vi "Data_2D_with_IgorX.vi"(6 "Data From Igor":bool, 8 "error in (no error)":errorcluster, 9 "Wave Name":string, 10 "Wave Prefix":string, 11 "2D Data IN":dbl[][](array[numeric])) -> (0 "error out":errorcluster, 2 "Wave Prefix Through":string, 3 "2D Data OUT":dbl[][](array[numeric]))   [LabVIEW 2014]
panel:
  in  "Igor Application IN":refnum<k7>
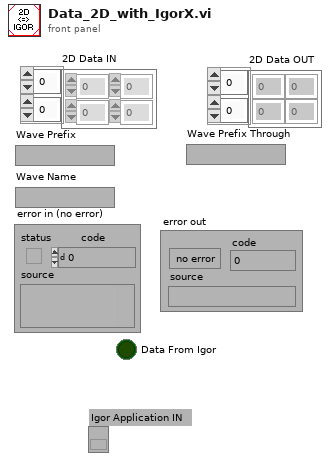
[diagram p1: front panel]
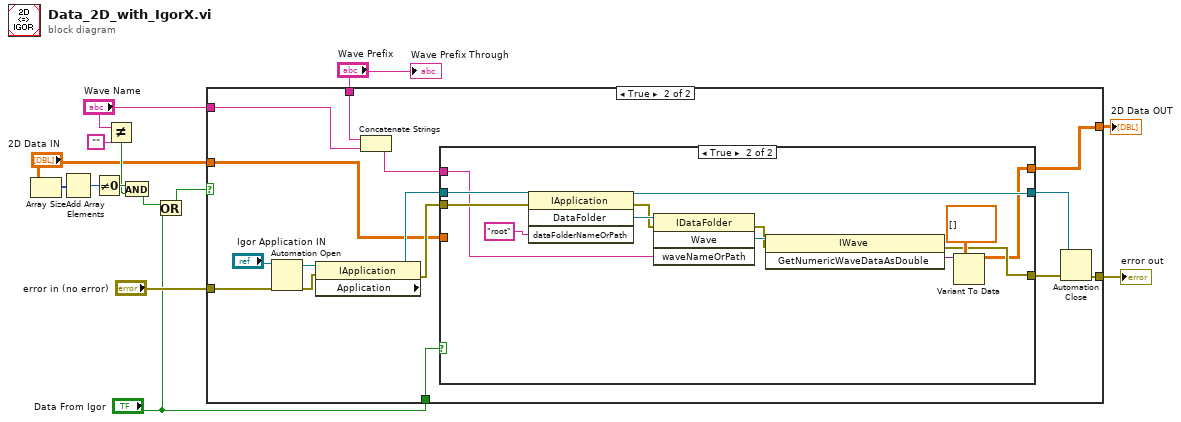
[diagram p0: block diagram]
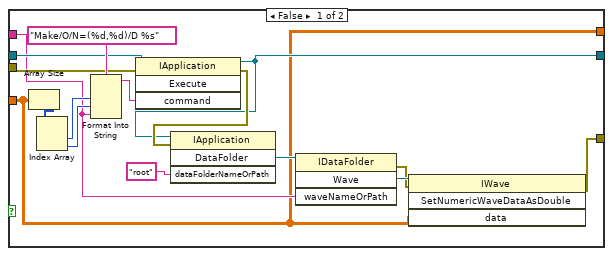
[diagram p3: hidden frame]
diagram:
  n1 = Array Size(array="2D Data IN") -> (size(s)=w14:i32[])
  n2 = Add Array Elements(numeric array=w14) -> (sum=w4:i32)
  n3 = Not Equal To 0?(x=w4) -> (x != 0?=w13:bool)
  n4 = Not Equal?(x="Wave Name", y="") -> (x != y?=w10:bool)
  n5 = And(x=w13, y=w10) -> (x .and. y?=w3:bool)
  n6 = Or(x=w3, y="Data From Igor") -> (x .or. y?=w1:bool)
  n7 = case shown="True" w1 {
    tunnel: "2D Data IN" -> [w15 w17]
    tunnel: "Wave Name" -> [_ w30]
    tunnel: "Wave Prefix" -> [_ w31]
    tunnel: "error in (no error)" -> [w16 w25]
    tunnel: [w16 w23] -> w8
    tunnel: "Data From Igor" -> [_ w29]
    tunnel: [w15 w18] -> w5
    frame False {
    }
    frame True {
      n8 = Automation Open(error in (no error)=w25, Automation Refnum="Igor Application IN") -> (Automation Refnum=w26:refnum<k7>, error out=w28:errorcluster)  [unwired: 2 in]
      n9 = property class="IApplication"(reference=w26, error in=w28) -> (error out=w24:errorcluster, "Application"=w22:refnum<k7>)  [unwired: 1 out]
      n10 = Concatenate Strings(w31, w30) -> (w20:string)
      n11 = case shown="True" w29 {
        tunnel: w24 -> [w45 w53]
        tunnel: [w37 w49] -> w21
        tunnel: w22 -> [w46 w52]
        tunnel: w20 -> [w33 w51]
        tunnel: [w38 w50] -> w19
        tunnel: [w32 w48] -> w18
        tunnel: w17 -> [w32 _]
        frame False {
          n12 = Array Size(array=w32) -> (size(s)=w36:i32[])
          n13 = Index Array(array=w36) -> (element #1=w35:i32, element #2=w34:i32)  [unwired: 2 in]
          n14 = Format Into String(format string="Make/O/N=(%d,%d)/D %s" ("dataFolderNameOrPath"), w35, w34, w33) -> (resulting string=w44:string)  [unwired: 2 in, 1 out]
          n15 = invoke class="IApplication" method="Execute"(reference=w46, error in=w45, "command"=w44) -> (reference out=w38:refnum<k7>, error out=w39:errorcluster)  [unwired: 1 in, 2 out]
          n16 = invoke class="IApplication" method="DataFolder"(reference=w38, error in=w39, "dataFolderNameOrPath"="root") -> ("DataFolder"=w40:refnum<k7>)  [unwired: 1 in, 3 out]
          n17 = invoke class="IDataFolder" method="Wave"(reference=w40, "waveNameOrPath"=w33) -> (error out=w41:errorcluster, "Wave"=w43:refnum<k7>)  [unwired: 2 in, 2 out]
          n18 = invoke class="IWave" method="SetNumericWaveDataAsDouble"(reference=w43, error in=w41, "data"=w32) -> (error out=w37:errorcluster)  [unwired: 1 in, 3 out]
        }
        frame True {
          n19 = invoke class="IApplication" method="DataFolder"(reference=w52, error in=w53, "dataFolderNameOrPath"="root") -> (reference out=w50:refnum<k7>, error out=w56:errorcluster, "DataFolder"=w57:refnum<k7>)  [unwired: 1 in, 1 out]
          n20 = invoke class="IDataFolder" method="Wave"(reference=w57, error in=w56, "waveNameOrPath"=w51) -> (error out=w58:errorcluster, "Wave"=w60:refnum<k7>)  [unwired: 1 in, 2 out]
          n21 = invoke class="IWave" method="GetNumericWaveDataAsDouble"(reference=w60, error in=w58) -> (error out=w49:errorcluster, "GetNumericWaveDataAsDouble"=w55:variant)  [unwired: 1 in, 1 out]
          n22 = Variant To Data(type=dbl[][] [] ("1D Data IN"), Variant=w55) -> (data=w48:dbl[][])  [unwired: 1 in, 1 out]
        }
      }
      n23 = Automation Close(3:w21, 5:w19) -> (0:w23:errorcluster)
    }
  }
  "error out" <- w8
  "2D Data OUT" <- w5
  "Wave Prefix Through" <- "Wave Prefix"
